vi "SDCP SMF Rx Logger - Test (version 1.1).vi"() -> ()   [LabVIEW 2020]
uses:
  Typedefs/SDCP SMF logger - SMF with timestamp.ctl
  Typedefs/SDCP - Serial Port Control - Commands.ctl
panel:
  out "Number of instantaeneous samples":i32
  out "Instantaeneous data":T1[](array[typedef])
  out "Elapse time (ms)":u32
  out "Logging started":bool
  out "Number of samples":i32
  in  "Number of iterations":i32
  in  "Log interval (ms)":u32
  in  "Stop logging":bool
  out "Rx data":T1[](array[typedef])
  in  "Baud rate":u32=9600
  in  "COM Port":refnum<visa-resource-name>
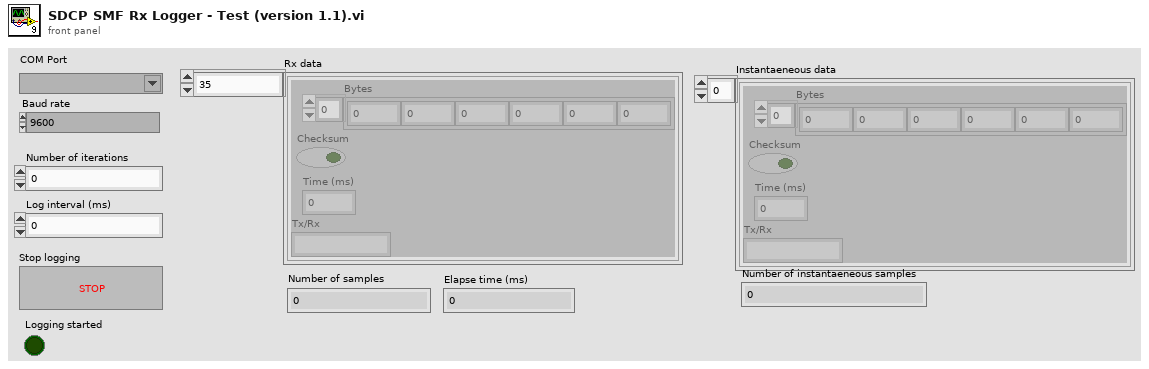
[diagram p1: front panel]
types:
  T1 = typedef "SDCP SMF logger - SMF with timestamp.ctl" = cluster{"Bytes":u8[], "Checksum":bool, "Time (ms)":u32, "Tx/Rx":string}
  T2 = enum16{"Start logging", "Get log data", "Stop logging"}
  T3 = typedef "SDCP - Serial Port Control - Commands.ctl" = enum16{"Open", "Read", "Write", "Get instance", "Close"}
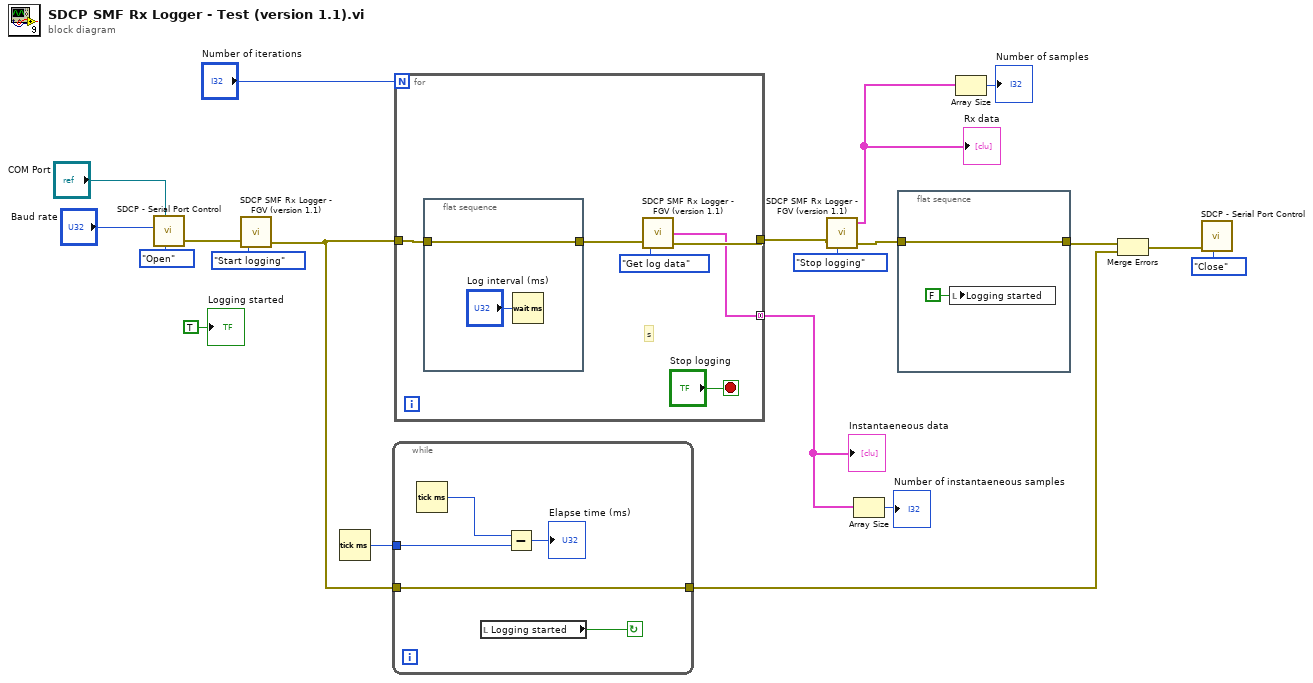
[diagram p0: block diagram]
diagram:
  n1 = call "SDCP - Serial Port Control.vi"("Command"=SDCP_-_Serial_Port_Control_-_Commands."Open", "VISA resource name"="COM Port", "Baud rate"="Baud rate") -> ("error out"=w18:errorcluster)  [unwired: 7 in, 1 out]
  n2 = call "SDCP SMF Rx Logger - FGV (version 1.1).vi"("Command"=T2."Start logging", "error in (no error)"=w18) -> ("error out"=w12:errorcluster)  [unwired: 2 out]
  n3 = Tick Count (ms)() -> (millisecond timer value=w6:u32)
  n4 = while {
    tunnel: w12 -> [w25]
    tunnel: [w25] -> w8
    tunnel: w6 -> [w23]
    stop <- w24 continue-if-true
    n5 = Tick Count (ms)() -> (millisecond timer value=w22:u32)
    n6 = local read "Logging started"() -> (w24:bool)
    n7 = Subtract(x=w22, y=w23) -> (x-y=→"Elapse time (ms)":u32)
  }
  n8 = for {
    N: "Number of iterations" -> [_]
    tunnel: w12 -> [w31]
    tunnel: [w28] -> w14
    tunnel: [w26] -> w2 mode=concatenating
    stop <- "Stop logging" stop-if-true
    # "s"
    n9 = flat-sequence {
      tunnel: w31 -> [w33]
      tunnel: [w33] -> w29
      frame #0 {
        n10 = Wait (ms)(milliseconds to wait="Log interval (ms)") -> ()  [unwired: 1 out]
      }
    }
    n11 = call "SDCP SMF Rx Logger - FGV (version 1.1).vi"("Command"=T2."Get log data", "error in (no error)"=w29) -> ("Instantaeneous data"=w26:T1[], "error out"=w28:errorcluster)  [unwired: 1 out]
  }
  "Instantaeneous data" <- w2
  n12 = call "SDCP SMF Rx Logger - FGV (version 1.1).vi"("Command"=T2."Stop logging", "error in (no error)"=w14) -> ("Logged data"=w5:T1[], "error out"=w10:errorcluster)  [unwired: 1 out]
  "Rx data" <- w5
  n13 = Array Size(array=w2) -> (size(s)=→"Number of instantaeneous samples":i32)
  n14 = flat-sequence {
    tunnel: w10 -> [w35]
    tunnel: [w35] -> w9
    frame #0 {
      n15 = local write "Logging started"(FALSE ("Logging started")) -> ()
    }
  }
  n16 = Array Size(array=w5) -> (size(s)=→"Number of samples":i32)
  n17 = Merge Errors(w9, w8) -> (w7:errorcluster)
  n18 = call "SDCP - Serial Port Control.vi"("Command"=SDCP_-_Serial_Port_Control_-_Commands."Close", "error in (no error)"=w7) -> ()  [unwired: 8 in, 2 out]
  "Logging started" <- TRUE ("Logging started")
